vi "test12.vi"() -> ()   [LabVIEW 2016]
panel:
  in  "G":u8
  in  "B":u8
  in  "R":u8
  out "Color":u32 format="%x"
  out "next 2":u16
  out "index 3":u16
  in  "reset 4":bool
  in  "doStep 2":bool=TRUE
  in  "maxCount 3":u16
  in  "reset 3":bool
  out "maxReached 2":bool
  out "index 2":u16
  in  "maxCount 2":u16
  out "minimum":i16
  in  "reset 2":bool
  in  "input":i16
  out "maxReachedBwd":bool
  out "indexBwd":u16
  out "nextBwd":u16
  out "next":u16
  out "index":u16
  out "maxReached":bool
  in  "reset":bool
  in  "doStep":bool=TRUE
  in  "start":u16
  in  "maxCount":u16
  in  "Tick":bool
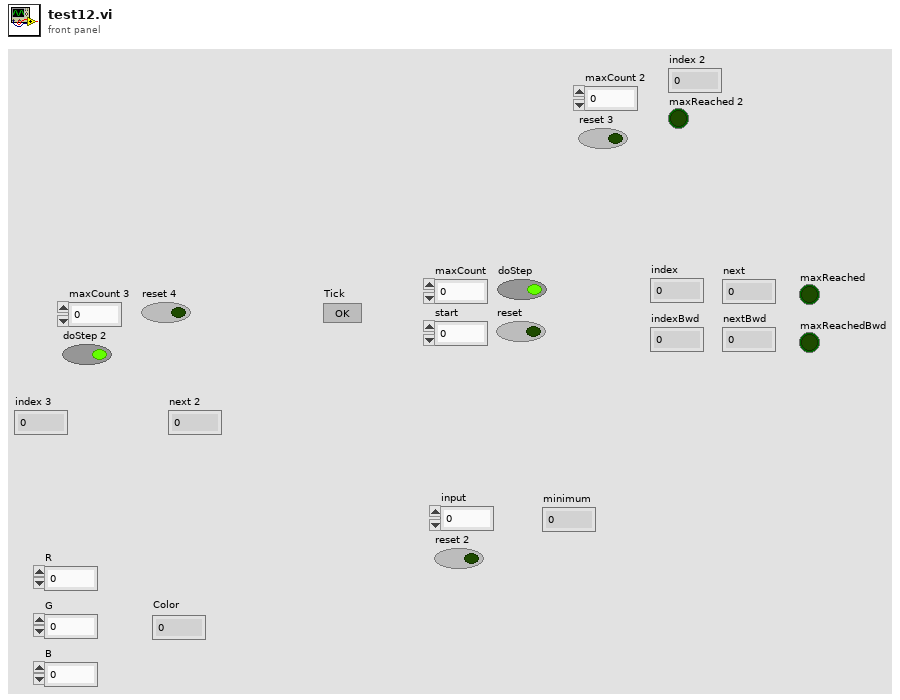
[diagram p1: front panel]
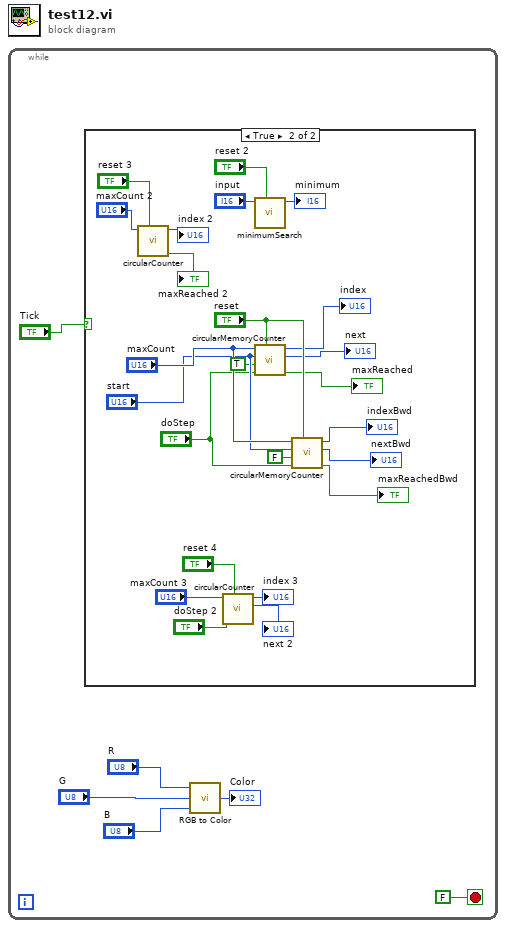
[diagram p0: block diagram]
diagram:
  n1 = while {
    stop <- FALSE stop-if-true
    n2 = case shown="True" "Tick" {
      frame False {
      }
      frame True {
        n3 = call "circularCounter.vi"("reset"="reset 3", "maxCount"="maxCount 2") -> ("maxReached"=→"maxReached 2":bool, "index"=→"index 2":u16)  [unwired: 7 in, 1 out]
        n4 = call "circularCounter.vi"("reset"="reset 4", "doStep"="doStep 2", "maxCount"="maxCount 3") -> ("next"=→"next 2":u16, "index"=→"index 3":u16)  [unwired: 6 in, 1 out]
        n5 = call "minimumSearch.vi"("reset"="reset 2", "input"="input") -> ("minimum"=→"minimum":i16)  [unwired: 9 in]
        n6 = call "circularMemoryCounter.vi"("reset"="reset", "doStep"="doStep", "foward"=TRUE, "start"="start", "maxCount"="maxCount") -> ("maxReached"=→"maxReached":bool, "next"=→"next":u16, "index"=→"index":u16)  [unwired: 4 in]
        n7 = call "circularMemoryCounter.vi"("reset"="reset", "doStep"="doStep", "foward"=FALSE, "start"="start", "maxCount"="maxCount") -> ("maxReached"=→"maxReachedBwd":bool, "next"=→"nextBwd":u16, "index"=→"indexBwd":u16)  [unwired: 4 in]
      }
    }
    n8 = call <vilib>:"RGB to Color.vi"("B"="B", "G"="G", "R"="R") -> ("Color"=→"Color":u32)
  }
